vi "temp.vi"() -> ()   [LabVIEW 2017]
uses:
  <vilib>/Instr/_visa.llb/VISA Configure Serial Port (Instr).vi
panel:
  out "UART Monitor (RX)":string
  in  "OK Button 2":bool
  in  "UART TX":string
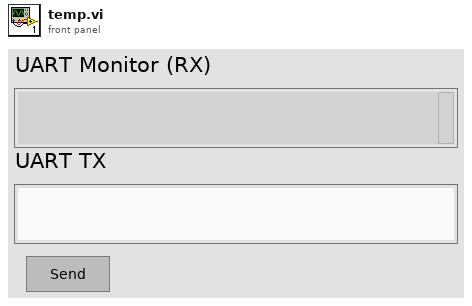
[diagram p1: front panel]
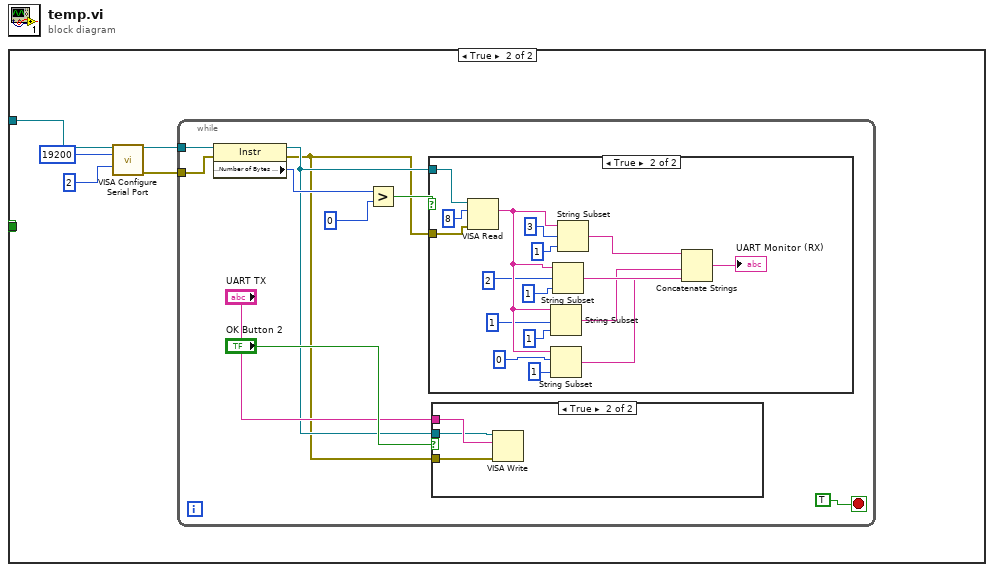
[diagram p0: block diagram]
diagram:
  n1 = case shown="True" {
    selector: _ -> [_ w2]
    tunnel: [_ w2] -> _
    tunnel: _ -> [_ w1]
    frame False {
    }
    frame True {
      n2 = call-poly "VISA Configure Serial Port"("VISA resource name"=w1, "baud rate (9600)"=19200, "parity (0:none)"=2) -> ("VISA resource name out"=w6:refnum<visa-resource-name>, "error out"=w5:errorcluster)  [unwired: 11 in]
      n3 = while {
        tunnel: w6 -> [w13]
        tunnel: w5 -> [w12]
        stop <- TRUE stop-if-true
        n4 = property class="Instr"(reference=w13, error in=w12) -> (reference out=w9:refnum<visa-resource-name>, error out=w8:errorcluster, "Serial Settings:Number of Bytes at Serial Port"=w16:u32)
        n5 = Greater?(x=w16, y=0) -> (0:w14:bool)
        n6 = case shown="True" w14 {
          tunnel: w9 -> [_ w35]
          tunnel: w8 -> [_ w34]
          frame False {
          }
          frame True {
            n7 = VISA Read(VISA resource name=w35, byte count=8, error in (no error)=w34) -> (read buffer=w24:string)  [unwired: 3 out]
            n8 = String Subset(string=w24, offset (0)=1, length (rest)=1) -> (substring=w30:string)
            n9 = String Subset(string=w24, offset (0)=0, length (rest)=1) -> (substring=w29:string)
            n10 = String Subset(string=w24, offset (0)=2, length (rest)=1) -> (substring=w31:string)
            n11 = String Subset(string=w24, offset (0)=3, length (rest)=1) -> (substring=w32:string)
            n12 = Concatenate Strings(w32, w31, w30, w29) -> (→"UART Monitor (RX)":string)
          }
        }
        n13 = case shown="True" "OK Button 2" {
          tunnel: "UART TX" -> [_ w19]
          tunnel: w9 -> [_ w18]
          tunnel: w8 -> [_ w17]
          frame False {
          }
          frame True {
            n14 = VISA Write(VISA resource name=w18, write buffer=w19, error in (no error)=w17) -> ()  [unwired: 3 out]
          }
        }
      }
    }
  }
